vi "XIPIN_Complex_Multiplier_6_0.vi"   [LabVIEW 2017]
doc: "Complex multiplication is a basic DSP operation. All operands, as well as the results, are represented as signed two's-complement data. Operand widths and result widths are parameterizable. Operand widths up to 63 bits are supported.\n------------------------------------\n<b>Need License</b> : No\n<b>Interface</b> : AXI4-Stream"
uses:
  <vilib>/rvi/XilinxIP/XIPIN_XNode/niFpgaXIPIN.xnode
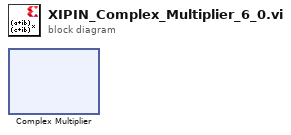
[diagram p0: block diagram]
diagram:
  n1 = xnode ("Complex Multiplier")() -> ()
